vi "Control_Fast_FID_Valve.vi"(3 "Mode":T5, 5 "Traverse line In":T2 {"Row Duration (mins)" format="%#.1f"; "Row No" min=0; "Trace Gas Concentration (%)" min=0.0 format="%#.2f"; "Emission Rate (l/min)" format="%#.2f"; "Tunnel Speed" format="%#.2f"; "Start X" format="%#.2f"; "Start Y" format="%#.2f"; "Start Z" format="%#.2f"; "End X" format="%#.2f"; "End Y" format="%#.2f"; "End Z" format="%#.2f"; "Averaging time (min)" min=0.0 format="%#.1f"}) -> (0 "Error Message":string, 1 "Status":T1, 2 "Traverse line Out":T2 {"Row Duration (mins)" format="%#.1f"; "Row No" min=0; "Trace Gas Concentration (%)" min=0.0 format="%#.2f"; "Emission Rate (l/min)" format="%#.2f"; "Tunnel Speed" format="%#.2f"; "Start X" format="%#.2f"; "Start Y" format="%#.2f"; "Start Z" format="%#.2f"; "End X" format="%#.2f"; "End Y" format="%#.2f"; "End Z" format="%#.2f"; "Averaging time (min)" min=0.0 format="%#.1f"})   [LabVIEW 2010]
uses:
  Gen Trav/Traverse_cluster.ctl
  Gen Trav/Spacing.ctl
  Controls/Multi_run_mode.ctl
  Controls/User_Specific_mode.ctl
  Gen Trav/Multi_Run_Status.ctl
panel:
  # "X           Y            Z"
  # "Start"
  # "End"
  # "X           Y            Z"
  # "Start"
  # "End"
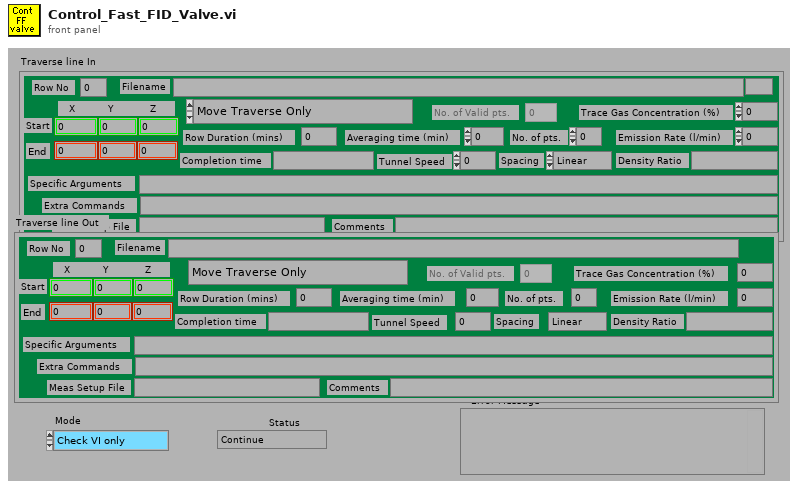
[diagram p1: front panel]
types:
  T1 = typedef "Multi_Run_Status.ctl" = enum16{"Continue", "Jump to Next Point", "Jump to Next Row", "Jump To Fall Back", "Terminate Run"}
  T2 = typedef "Traverse_cluster.ctl" = cluster{"Start X":dbl, "Start Y":dbl, "Start Z":dbl, "End X":dbl, "End Y":dbl, "End Z":dbl, "No. of pts.":i32, "Spacing":T3, "Filename":path, "Tunnel Speed":dbl, "Averaging time (min)":dbl, "Extra Commands":string, "Specific Arguments":string, "Emission Rate (l/min)":dbl, "Trace Gas Concentration (%)":dbl, "Density Ratio":string, "Comments":string, "Row No":i32, "Row Type Selector":T4, "Completion time":string, "Row Duration (mins)":dbl, "No. of Valid pts.":i32, "Meas Setup File":string}
  T3 = typedef "Spacing.ctl" = enum16{"Linear", "Log", "Gauss", "Specified", "N/A"}
  T4 = typedef "Multi_run_mode.ctl" = enum16{"Move Traverse Only", "Set Tunnel Speed Only", "Set Source Only", "Set Measurement Conditions", "Single Measurement", "Vertical Profile", "Lateral Profile", "Longitudinal Profile", "Explore Volume", "Multi-Axis Profile", "Auto Calibrate", "Meas Fast FID Bkgnd", "Check Beam Power", "Scanning Valve Measurement", "Run VI Named:", "Set ADAM Ch", "Wait (minutes)", "Send Message", "Synchronize With:", "Fall Back to this Row", "Turn Off Row Repeating", "Blank Row"}
  T5 = typedef "User_Specific_mode.ctl" = enum16{"Check VI only", "Run VI"}
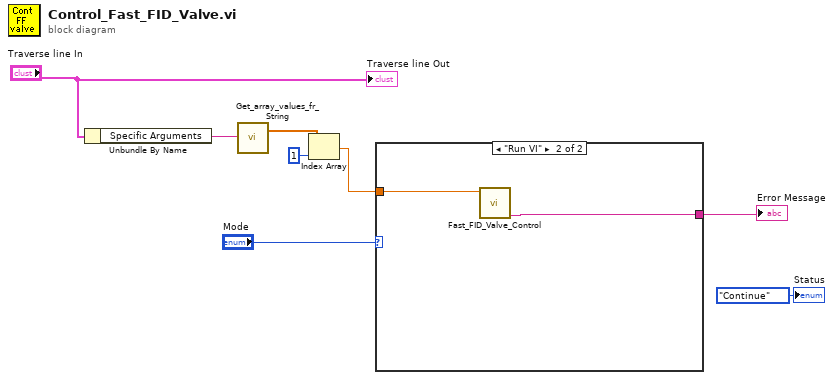
[diagram p0: block diagram]
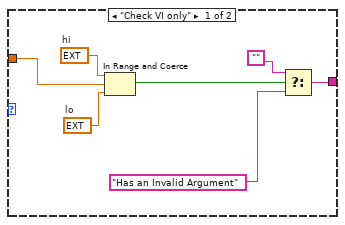
[diagram p2: hidden frame]
diagram:
  n1 = Unbundle By Name("Traverse line In") -> ("Specific Arguments"=w2:string)
  n2 = call "Get_array_values_fr_String.vi"("String Value"=w2) -> ("Numeric Array"=w4:dbl[])  [unwired: 1 out]
  n3 = Index Array(array=w4, index=1 ("Index")) -> (element=w6:dbl)
  n4 = case shown="\"Run VI\"" "Mode" {
    tunnel: w6 -> [w15 w17]
    tunnel: [w11 w16] -> w5
    frame "Check VI only" {
      w13 = ext 0.8  # lo
      w14 = ext 4.1  # hi
      n5 = In Range and Coerce(upper limit=w14, x=w15, lower limit=w13) -> (In Range?=w12:bool)  [unwired: 1 out]
      n6 = Select(t="", s=w12, f="Has an Invalid Argument") -> (s? t:f=w11:string)
    }
    frame "Run VI" {
      n7 = call "Fast_FID_Valve_Control.vi"("Requested Position"=w17) -> ("Error Message"=w16:string)  [unwired: 6 out]
    }
  }
  "Error Message" <- w5
  "Traverse line Out" <- "Traverse line In"
  "Status" <- Multi_Run_Status."Continue" ("Status")
